vi "command_subscriber.vi"() -> ()   [LabVIEW 2016]
uses:
  ts_sallv_exa/DataTypes/command_start.ctl
  ts_sallv_exa/DataTypes/ackcmd.ctl
  ts_sallv_exa/SALLV_EXA.lvlib
panel:
  out "command_start_Ctl out":T1
  out "Stop":bool=TRUE
  in  "stop":bool
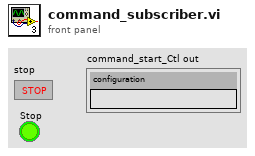
[diagram p1: front panel]
types:
  T1 = typedef "SALLV_EXA.lvlib/command_start.ctl" = cluster{"configuration":string}
  T2 = typedef "SALLV_EXA.lvlib/ackcmd.ctl" = cluster{"cmdSeqNum":i32, "ack":i32, "error":i32, "result":string}
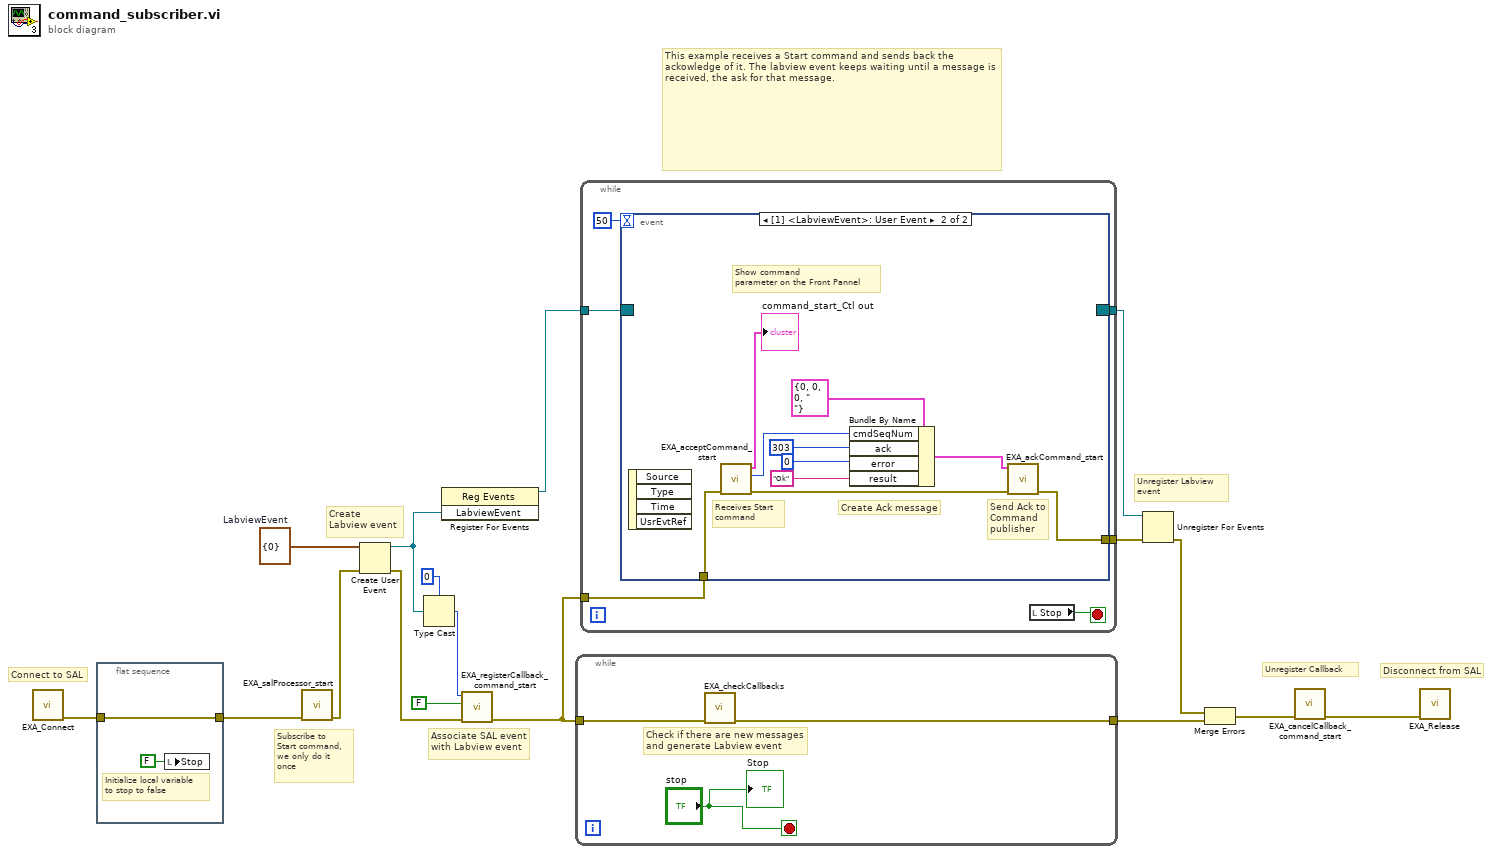
[diagram p0: block diagram]
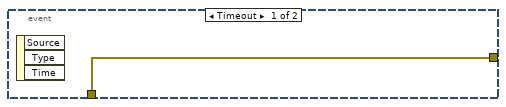
[diagram p2: hidden frame]
diagram:
  w14 = cluster{"Data":i32} {"Data"=0}  # LabviewEvent
  # "This example receives a Start command and sends back the ackowledge of it. The labview event keeps waiting until a message is received, the ask for that message."
  # "Unregister Labview\nevent"
  # "Create Labview event"
  # "Associate SAL event\nwith Labview event"
  # "Unregister Callback"
  # "Subscribe to \nStart command,\nwe only do it \nonce"
  # "Disconnect from SAL"
  # "Connect to SAL"
  n1 = call "EXA_Connect.vi"() -> ("error out"=w16:errorcluster)  [unwired: 10 in, 1 out]
  n2 = flat-sequence {
    tunnel: w16 -> [w18]
    tunnel: [w18] -> w15
    frame #0 {
      # "Initialize local variable \nto stop to false"
      n3 = local write "Stop"(FALSE ("Stop")) -> ()
    }
  }
  n4 = call "EXA_salProcessor_start.vi"("error in (no error)"=w15) -> ("error out"=w13:errorcluster)  [unwired: 9 in, 1 out]
  n5 = Create User Event(user event datatype=w14, error in=w13) -> (user event=w11:refnum<user-event>, error out=w12:errorcluster)
  n6 = Type Cast(type=0 ("handle"), x=w11) -> (*(type *) &x=w9:i32)
  n7 = register-events(w11) -> (reference out=w8:refnum<event-registration>)  [unwired: 2 in, 1 out]
  n8 = call "EXA_registerCallback_command_start.vi"("error in (no error)"=w12, "skipOld"=FALSE, "handle"=w9) -> ("error out"=w6:errorcluster)  [unwired: 7 in, 1 out]
  n9 = while {
    tunnel: w6 -> [w21]
    tunnel: [w20] -> w5
    stop <- "stop" stop-if-true
    # "Check if there are new messages \nand generate Labview event"
    n10 = call "EXA_checkCallbacks.vi"("error in (no error)"=w21) -> ("error out"=w20:errorcluster)  [unwired: 10 in]
    "Stop" <- "stop"
  }
  n11 = while {
    tunnel: w8 -> [w26]
    tunnel: w6 -> [w25]
    tunnel: [w24] -> w3
    tunnel: [w23] -> w2
    stop <- w28 stop-if-true
    n12 = event shown="[1] <LabviewEvent>: User Event" {
      selector: w26 -> [_ _]
      dyn-events: [_ _] -> w23
      timeout: 50 -> [_ _]
      tunnel: w25 -> [w29 w39]
      tunnel: [w29 w38] -> w24
      event Timeout {
        n13 = event-data() -> ()  [unwired: 1 in, 3 out]
      }
      event User Event {
        # "Create Ack message"
        # "Show command \nparameter on the Front Pannel"
        # "Send Ack to\nCommand \npublisher"
        # "Receives Start\ncommand"
        n14 = event-data() -> ()  [unwired: 1 in, 4 out]
        n15 = call "EXA_acceptCommand_start.vi"("error in (no error)"=w39) -> ("error out"=w37:errorcluster, "function return"=w30:i32, "command_start_Ctl out"=→"command_start_Ctl out":T1)  [unwired: 8 in]
        n16 = Bundle By Name(cluster=T2 {"cmdSeqNum"=0, "ack"=0, "error"=0, "result"="                                                                                                                                                                                                                                                                "} ("ackcmd_Ctl"), "cmdSeqNum"=w30, "ack"=303, "error"=0, "result"="Ok") -> (w34:T2)
        n17 = call "EXA_ackCommand_start.vi"("error in (no error)"=w37, "ackcmd_Ctl"=w34) -> ("error out"=w38:errorcluster)  [unwired: 7 in, 2 out]
      }
    }
    n18 = local read "Stop"() -> (w28:bool)
  }
  n19 = Unregister For Events(event registration refnum=w2, error in=w3) -> (error out=w1:errorcluster)
  n20 = Merge Errors(w1, w5) -> (w4:errorcluster)
  n21 = call "EXA_cancelCallback_command_start.vi"("error in (no error)"=w4) -> ("error out"=w7:errorcluster)  [unwired: 9 in, 1 out]
  n22 = call "EXA_Release.vi"("error in (no error)"=w7) -> ()  [unwired: 9 in, 2 out]
